vi "Battery - myRIO verB.vi"(8 "Error input":errorcluster, 10 "Command to write":string(combo)="RD_STAT>\r", 11 "VISA resource name out":refnum<visa-resource-name>) -> (0 "Error Out":errorcluster, 1 "Read Buffer":string, 2 "csv output":string, 3 "OUTPUT":string[](array[string]))   [LabVIEW 2015]
doc: "This VI is going to work into myRIO and has three sections:\n\n1. Take data from the Charging Regulator.\n2. Fitting the discharge/charge curve and calculate the SoC (State of Charge).\n3. Publish the data, included SoC, into the MQTT Broker, using Internet connection."
panel:
  out "Fitting values":T1 {"Times" format="%#_13g"}
  in  "?":T2 {"Time" format="%#_13g"}
  out "State if not Fit":string
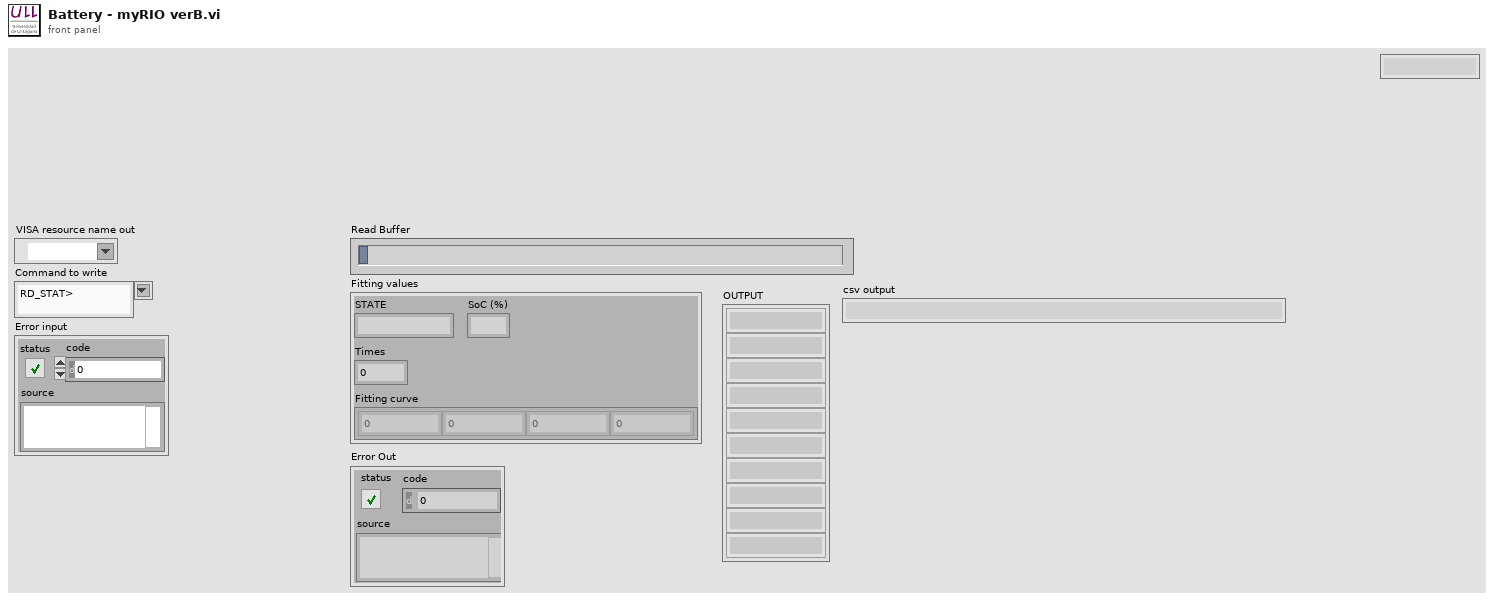
[diagram p1: front panel]
types:
  T1 = cluster{"STATE":string, "Times":dbl, "Fitting curve":dbl[], "SoC (%)":string}
  T2 = cluster{"STATE":string, "Time":dbl, "Curve":dbl[], "SoC (%)":string}
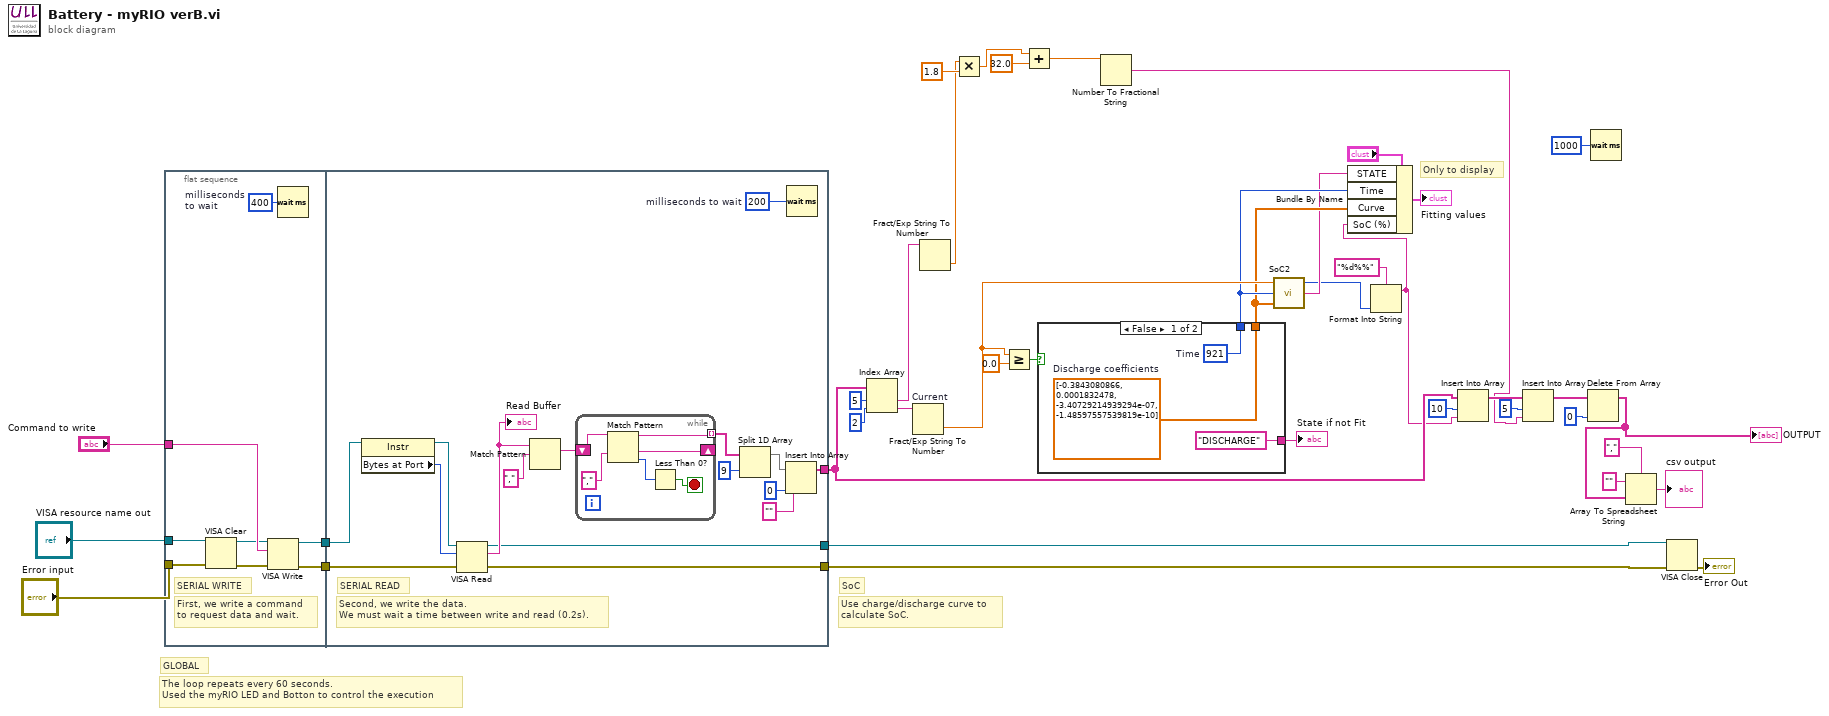
[diagram p0: block diagram]
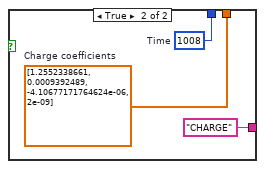
[diagram p2: hidden frame]
diagram:
  # "Only to display"
  # "Use charge/discharge curve to\ncalculate SoC."
  # "SoC"
  # "The loop repeats every 60 seconds.\nUsed the myRIO LED and Botton to control the execution"
  # "GLOBAL"
  n1 = flat-sequence {
    tunnel: "VISA resource name out" -> [w47]
    tunnel: "Error input" -> [w46]
    tunnel: "Command to write" -> [w45]
    tunnel: [w49] -> w37
    tunnel: [w48] -> w36
    tunnel: [w52] -> w39
    tunnel: w37 -> [w53]
    tunnel: w36 -> [w52]
    tunnel: [w51] -> w38
    tunnel: [w50] -> w30
    frame #0 {
      w44 = u32 400  # milliseconds to wait
      # "First, we write a command\nto request data and wait."
      # "SERIAL WRITE"
      n2 = VISA Clear(VISA resource name=w47, error in (no error)=w46) -> (VISA resource name out=w43:refnum<visa-resource-name>, error out=w42:errorcluster)
      n3 = VISA Write(VISA resource name=w43, write buffer=w45, error in (no error)=w42) -> (VISA resource name out=w49:refnum<visa-resource-name>, error out=w48:errorcluster)  [unwired: 1 out]
      n4 = Wait (ms)(milliseconds to wait=w44) -> ()  [unwired: 1 out]
    }
    frame #1 {
      w62 = u32 200  # milliseconds to wait
      # "Second, we write the data.\nWe must wait a time between write and read (0.2s)."
      # "SERIAL READ"
      n5 = property class="Instr"(reference=w53) -> (reference out=w64:refnum<visa-resource-name>, "Bytes at Port"=w63:u32)  [unwired: 1 in, 1 out]
      n6 = VISA Read(VISA resource name=w64, byte count=w63, error in (no error)=w52) -> (VISA resource name out=w51:refnum<visa-resource-name>, read buffer=w57:string)  [unwired: 2 out]
      "Read Buffer" <- w57
      n7 = Match Pattern(string=w57, regular expression=",") -> (after substring=w60:string)  [unwired: 1 in, 3 out]
      n8 = while {
        tunnel: [w67] -> w58 mode=indexing
        shift-right: [w68] -> _
        shift-left: w60 -> [w70]
        stop <- w65 stop-if-true
        n9 = Match Pattern(string=w70, regular expression=",") -> (before substring=w67:string, after substring=w68:string, offset past match=w66:i32)  [unwired: 2 out]
        n10 = Less Than 0?(x=w66) -> (x < 0?=w65:bool)
      }
      n11 = Split 1D Array(array=w58, index=9) -> (first subarray=w54:string[])  [unwired: 1 out]
      n12 = Insert Into Array(array=w54, index=0, new element="" ("new element/subarray")) -> (w50:string[])
      n13 = Wait (ms)(milliseconds to wait=w62) -> ()  [unwired: 1 out]
    }
  }
  n14 = Index Array(array=w30, index #1=5 ("index"), index #2=2 ("index")) -> (element #1=w5:string, element #2=w32:string)
  n15 = Fract/Exp String To Number "Current"(string=w32) -> (number=w15:dbl)  [unwired: 3 in, 1 out]
  n16 = Fract/Exp String To Number(string=w5) -> (number=w4:dbl)  [unwired: 3 in, 1 out]
  n17 = Multiply(x=w4, y=1.8) -> (x*y=w3:dbl)
  n18 = Greater Or Equal?(x=w15, y=0.0 ("x")) -> (x >= y?=w26:bool)
  n19 = Add(x=w3, y=32.0) -> (x+y=w2:dbl)
  n20 = case shown="False" w26 {
    tunnel: [w72 w75] -> w13
    tunnel: ["DISCHARGE" "CHARGE"] -> w25
    tunnel: [w71 w74] -> w14
    frame False {
      w71 = 921  # Time
      w72 = dbl[] [-0.3843080866, 0.0001832478, -3.40729214939294e-07, -1.48597557539819e-10]  # Discharge coefficients
    }
    frame True {
      w74 = 1008  # Time
      w75 = dbl[] [1.2552338661, 0.0009392489, -4.10677171764624e-06, 2e-09]  # Charge coefficients
    }
  }
  "State if not Fit" <- w25
  n21 = Number To Fractional String(number=w2) -> (F-format string=w1:string)  [unwired: 3 in]
  n22 = call "SoC2.vi"("Coefficients"=w13, "Time"=w14, "BAT Current (A)"=w15) -> ("State"=w12:string, "SoC (%)"=w11:i32)  [unwired: 1 out]
  n23 = Format Into String(format string="%d%%", w11) -> (resulting string=w23:string)  [unwired: 2 in, 1 out]
  n24 = Bundle By Name(cluster="?", "STATE"=w12, "Time"=w14, "Curve"=w13, "SoC (%)"=w23) -> (→"Fitting values":T2)
  n25 = Insert Into Array(array=w30, index=10, new element=w23) -> (w8:string[])
  n26 = Insert Into Array(array=w8, index=5, new element=w1) -> (w7:string[])
  n27 = Delete From Array(array=w7, index=0) -> (array with subset deleted=w19:string[])  [unwired: 1 in, 1 out]
  "OUTPUT" <- w19
  n28 = Wait (ms)(milliseconds to wait=u32 1000) -> ()  [unwired: 1 out]
  n29 = Array To Spreadsheet String(delimiter (Tab)=",", array=w19, 3:"" ("format string")) -> (spreadsheet string=→"csv output":string)
  n30 = VISA Close(VISA resource name=w38, error in (no error)=w39) -> (error out=→"Error Out":errorcluster)
